vi "CreateSession.vi"(8 "error in (no error)":errorcluster, 11 "ONNX model path":path) -> (0 "error out":errorcluster, 3 "session id out":i32)   [LabVIEW 2017, in "libonnx_wrapper.lvlib"]
doc: "* @brief Создать новую сессию и загрузить ONNX модель в память\n * \n * Эта функция выделяет уникальный SessionID, загружает модель из файла,\n * анализирует её структуру (входы, выходы, типы данных, формы тензоров)\n * и сохраняет всю информацию для последующего использования.\n * \n * @param modelPath [IN] Путь к файлу модели в формате .onnx (абсолютный или относительный)\n * \n * @return int32: SessionID (положительное целое число >= 1) при успехе\n * @return int32: -1 при ошибке (неверный путь, повреждённая модель, нехватка памяти)\n * \n * @note SessionID необходимо сохранить и передавать во все последующие функции\n * @note При ошибке сессия автоматически удаляется из внутреннего хранилища\n */\nint CreateSession(const char* modelPath);"
uses:
  libonnx_wrapper.lvlib
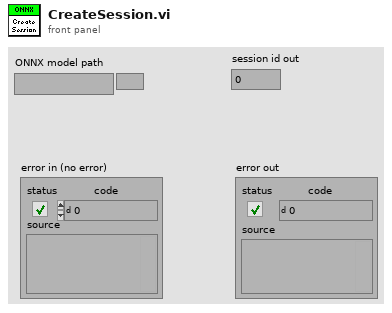
[diagram p1: front panel]
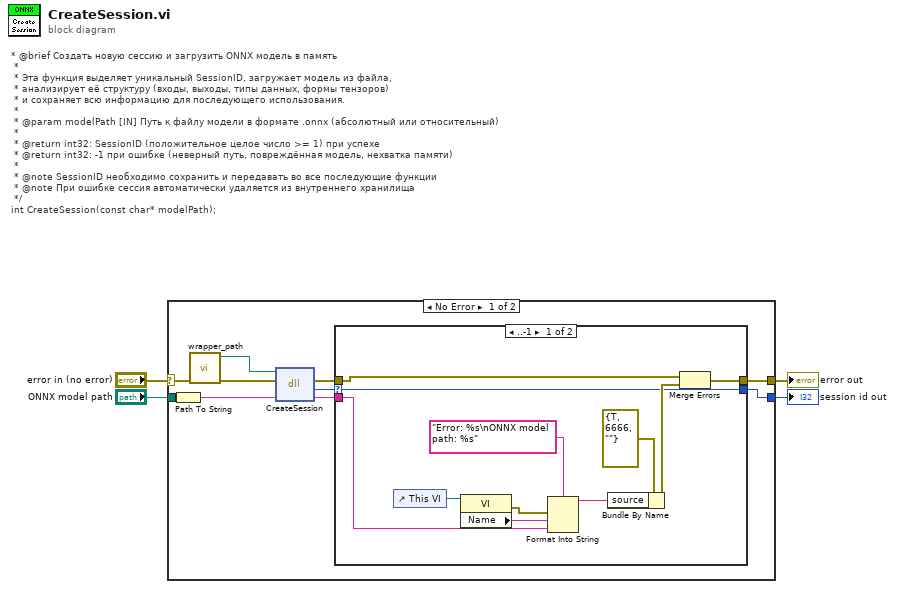
[diagram p0: block diagram]
diagram:
  # "* @brief Создать новую сессию и загрузить ONNX модель в память\n * \n * Эта функция выделяет уникальный SessionID, загружает модель из файла,\n * анализирует её структуру (входы, выходы, типы данных, формы тензоров)\n * и сохраняет всю информацию для последующего использования.\n * \n * @param modelPath [IN] Путь к файлу модели в формате .onnx (абсолютный или относительный)\n * \n * @return int32: SessionID (положительное целое число >= 1) при успехе\n * @return int32: -1 при ошибке (неверный путь, повреждённая модель, нехватка памяти)\n * \n * @note SessionID необходимо сохранить и передавать во все последующие функции\n * @note При ошибке сессия автоматически удаляется из внутреннего хранилища\n */\nint CreateSession(const char* modelPath);"
  n1 = case shown="No Error" "error in (no error)" {
    selector: "error in (no error)" -> [w5 w28]
    tunnel: "ONNX model path" -> [w14 _]
    tunnel: [w8 _] -> w3
    tunnel: [w7 w28] -> w2
    frame No Error {
      n2 = Path To String(path=w14) -> (string=w13:string)
      n3 = call "wrapper_path.vi"("error in (no error)"=w5) -> ("error out"=w12:errorcluster, "wrapper path"=w11:path)  [unwired: 9 in]
      n4 = dll-call lib="home/ivan/LabVIEWData/ONNX/Test/libonnx_wrapper/unix64/libonnx_wrapper.so" fn="CreateSession"(path in=w11, error in=w12, "modelPath"=w13) -> (error out=w10:errorcluster, "return"=w9:i32, "modelPath"=w6:string)  [unwired: 1 in, 1 out]
      n5 = case shown="..-1" w9 {
        selector: w9 -> [w15 w26]
        tunnel: w10 -> [w17 w27]
        tunnel: [w18 w27] -> w7
        tunnel: w6 -> [w16 _]
        tunnel: [w15 w26] -> w8
        frame ..-1 {
          n6 = control-ref of="This VI"() -> (w22:refnum<vi>)
          n7 = property class="VI"(reference=w22) -> (error out=w19:errorcluster, "Name"=w21:string)  [unwired: 1 in, 1 out]
          n8 = Format Into String(format string="Error: %s\nONNX model path: %s", error in=w19, w21, w16) -> (resulting string=w23:string)  [unwired: 1 in, 1 out]
          n9 = Bundle By Name(cluster=errorcluster {"status"=TRUE, "code"=6666, "source"=""} ("error out"), "source"=w23) -> (w24:errorcluster)
          n10 = Merge Errors(w17, w24) -> (w18:errorcluster)
        }
        frame 0.. {
        }
      }
    }
    frame Error {
    }
  }
  "session id out" <- w3
  "error out" <- w2
